vi "Write TaskConfig.vi"(8 "error in (no error)":errorcluster, 10 "TaskConfig":T1={"Drive"=enum."NI_DAQmx", "TaskType"=enum."AI", "PhysicalChannels"="", "SampleRateConfiguration"={"SampleRate"=0.0, "SamplesPerChannel"=0, "SamplesPerRead"=0, "SampleMode"=10123, "Clock Source"="OnboardClock"}, "ChannelConfig"={}, "Enable"=FALSE, "ShowPanel"=FALSE} {"SampleRateConfiguration"."SampleMode" items=["Finite Samples"=10178, "Continuous Samples"=10123, "Hardware Timed Single Point"=12522]}, 11 "AI_Task in":refnum<class "AI_Task.lvclass">) -> (0 "error out":errorcluster, 3 "AI_Task out":refnum<class "AI_Task.lvclass">)   [LabVIEW 2025, in "AI_Task.lvlib" / "AI_Task.lvclass"]
uses:
  AI_Task.lvclass
  AI_Task.lvclass/AI_Task.ctl
  DAQ_Module/DAQ_Module/DAQ_Module/DAQ_AI_Task_Config.ctl
  DAQ_Module/DAQ_Module/DAQ_Module/DAQ_Module.lvclass
  Waveform_Task/Waveform_Task/Waveform_Task.lvclass
  DAQ_Module/DAQ_Module/DAQ_Module/DAQ_Task_Type.ctl
  DAQ_Module/DAQ_Module/DAQ_Module/DAQ_Task_Config.ctl
  DAQ_Module/DAQ_Module/DAQ_Module/DAQ_HW_Type.ctl
  DAQ_Module/DAQ_Module/DAQ_Module/DAQ_SampleRateConfig.ctl
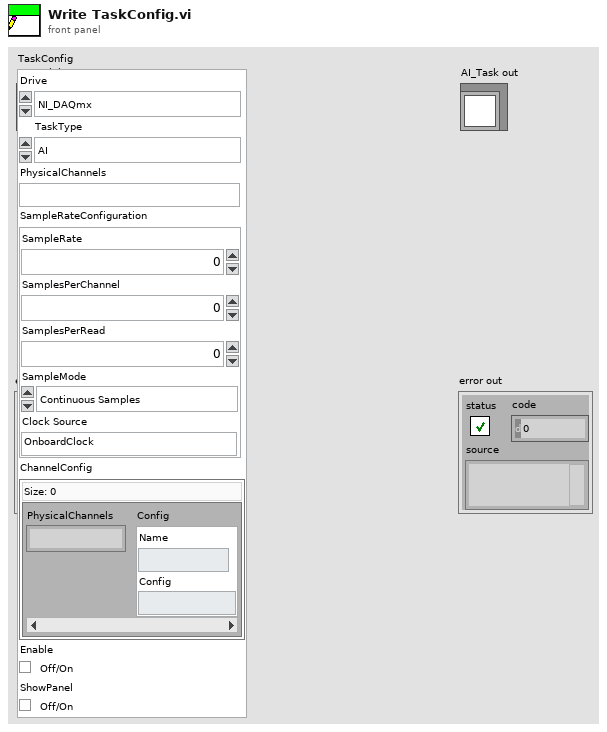
[diagram p1: front panel]
types:
  T1 = typedef "DAQ_Module.lvlib/DAQ_Module.lvclass/DAQ_Task_Config.ctl" = cluster{"Drive":T2, "TaskType":T3, "PhysicalChannels":string, "SampleRateConfiguration":T4, "ChannelConfig":map{string, cluster{"Name":string, "Config":string}}, "Enable":bool, "ShowPanel":bool}
  T2 = typedef "DAQ_Module.lvlib/DAQ_Module.lvclass/DAQ_HW_Type.ctl" = enum16{"NI_DAQmx", "Simulated_DAQ"}
  T3 = typedef "DAQ_Module.lvlib/DAQ_Module.lvclass/DAQ_Task_Type.ctl" = enum16{"AI", "Linear", "Angular", "AO"}
  T4 = typedef "DAQ_Module.lvlib/DAQ_Module.lvclass/DAQ_SampleRateConfig.ctl" = cluster{"SampleRate":dbl, "SamplesPerChannel":u32, "SamplesPerRead":i32, "SampleMode":i32, "Clock Source":string}
  T5 = typedef "DAQ_Module.lvlib/DAQ_Module.lvclass/DAQ_AI_Task_Config.ctl" = cluster{"MaxValue":dbl, "MinValue":dbl, "InputTerminalConfiguration":i32}
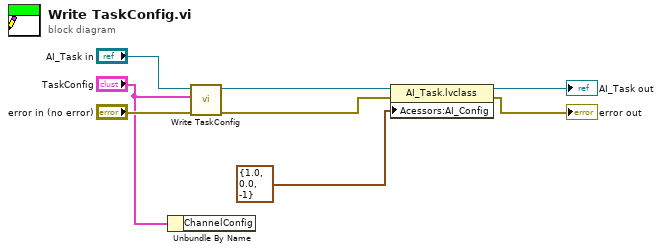
[diagram p0: block diagram]
diagram:
  n1 = Unbundle By Name("TaskConfig") -> ()  [unwired: 1 out]
  n2 = call-parent "Write TaskConfig.vi"("error in (no error)"="error in (no error)", "TaskConfig"="TaskConfig", "Task_Abstr in"="AI_Task in") -> ("error out"=w3:errorcluster, "Task_Abstr out"=w8:refnum<class "AI_Task.lvclass">)  [unwired: 7 in]
  n3 = property class="AI_Task.lvclass"(reference=w8, error in=w3, "Acessors:AI_Config"=T5 {"MaxValue"=1.0, "MinValue"=0.0, "InputTerminalConfiguration"=-1} ("AI_Config")) -> (reference out=→"AI_Task out":refnum<class "AI_Task.lvclass">, error out=→"error out":errorcluster)
